vi "test_LoadCommandlineArgs_AddPackedLibMissingPath.vi"() -> (3 "Pass?":bool)   [LabVIEW 2019, in "Tests.SolutionBuilder.lvlib"]
uses:
  Tests.SolutionBuilder.lvlib
  SolutionBuilder/Community/Options.ctl
  SolutionBuilder/SolutionBuilder.lvclass
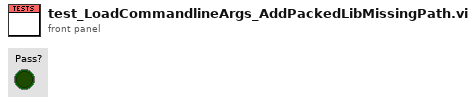
[diagram p1: front panel]
types:
  T1 = typedef "SolutionBuilder.lvlib/SolutionBuilder.lvclass/Options.ctl" = cluster{"Path":path, "Preview?":bool, "Quiet?":bool, "Log file":path, "Success file":path, "Rebuild?":bool, "Keep split projects?":bool, "Version string":string}
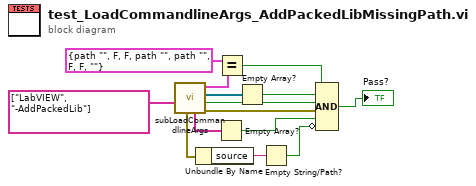
[diagram p0: block diagram]
diagram:
  n1 = call "subLoadCommandlineArgs.vi"("App.Args"=string[] ["LabVIEW", "-AddPackedLib"]) -> ("error out"=w12:errorcluster, "From command line?"=w6:bool, "Pre-built libraries"=w9:refnum<class "ProjectItem.lvclass">[], "Options"=w10:T1, "Active targets"=w5:string[], "warnings out"=w4:errorcluster)  [unwired: 5 in]
  n2 = Unbundle By Name(w4) -> ("source"=w3:string)
  n3 = Empty Array?(array=w5) -> (empty?=w1:bool)
  n4 = Equal?(x=T1 {"Path"=path "", "Preview?"=FALSE, "Quiet?"=FALSE, "Log file"=path "", "Success file"=path "", "Rebuild?"=FALSE, "Keep split projects?"=FALSE, "Version string"=""} ("Options"), y=w10) -> (x = y?=w7:bool)
  n5 = Empty Array?(array=w9) -> (empty?=w8:bool)
  n6 = Empty String/Path?(string/path=w3) -> (empty?=w2:bool)
  n7 = Compound Arithmetic op=AND(w7, w8, w6, w12, w1, invert w2) -> (→"Pass?":bool)
